vi "Get Step Size Level Amplitude.vi"(8 "error in (no error)":errorcluster, 10 "Output BNC (T0)":T1 items=["T0", "AB", "CD", "EF", "GH"], 11 "VISA resource name":refnum<visa-resource-name>) -> (0 "error out":errorcluster, 2 "Step Size Level Amplitue [V]":dbl, 3 "VISA resource name out":refnum<visa-resource-name>, 4 "Device Errors":cluster{"code":i32, "Text":string}[](array[cluster]))   [LabVIEW 2014, in "Stanford Research DG645 - Driver.lvlib"]
doc: "Delay and Output Command: SSLA? b\nInstrument Error Check\n\nQuery current step size of the level amplitude (in volt) for output b."
uses:
  Stanford Research DG645 - Driver.lvlib
  Output BNC.ctl
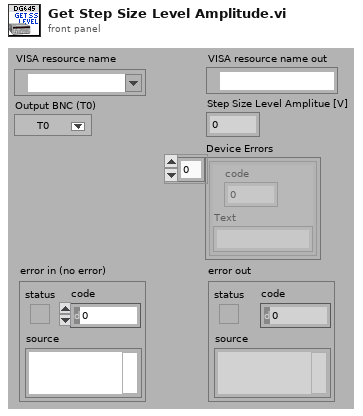
[diagram p1: front panel]
types:
  T1 = typedef "Stanford Research DG645 - Driver.lvlib/Output BNC.ctl" = i32
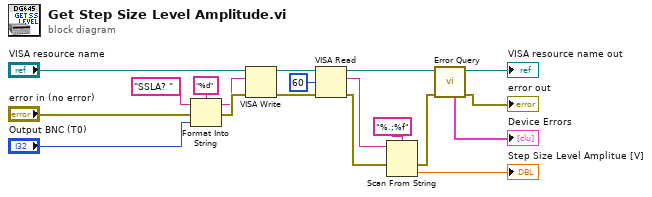
[diagram p0: block diagram]
diagram:
  n1 = Format Into String(format string="%d", initial string="SSLA? " ("command"), error in="error in (no error)", "Output BNC (T0)") -> (resulting string=w15:string, error out=w16:errorcluster)
  n2 = VISA Write(VISA resource name="VISA resource name", write buffer=w15, error in (no error)=w16) -> (VISA resource name out=w12:refnum<visa-resource-name>, error out=w11:errorcluster)  [unwired: 1 out]
  n3 = VISA Read(VISA resource name=w12, byte count=u32 60, error in (no error)=w11) -> (VISA resource name out=w10:refnum<visa-resource-name>, read buffer=w7:string, error out=w3:errorcluster)  [unwired: 1 out]
  n4 = Scan From String(format string="%.;%f", input string=w7, error in=w3) -> (error out=w2:errorcluster, output 1=→"Step Size Level Amplitue [V]":dbl)  [unwired: 2 in, 2 out]
  n5 = call "Error Query.vi"("error in (no error)"=w2, "VISA resource name"=w10) -> ("error out"=→"error out":errorcluster, "VISA resource name out"=→"VISA resource name out":refnum<visa-resource-name>, "Device Errors"=→"Device Errors":cluster{"code":i32, "Text":string}[])  [unwired: 7 in]
